vi "process_resistance_arrays.vi"(8 "error in (no error)":errorcluster, 10 "Array":dbl[][](array[numeric]), 11 "TempProbeSet in":refnum<class "TempProbeSet.lvclass">) -> (0 "error out":errorcluster, 3 "TempProbeSet out":refnum<class "TempProbeSet.lvclass">)   [LabVIEW 2010, in "TempProbeSet.lvclass"]
uses:
  TempProbeSet.lvclass
  TempProbe.lvclass
  accessors/read_probes.vi
  accessors/write_probes.vi
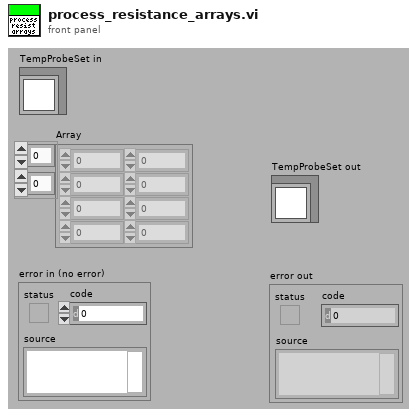
[diagram p1: front panel]
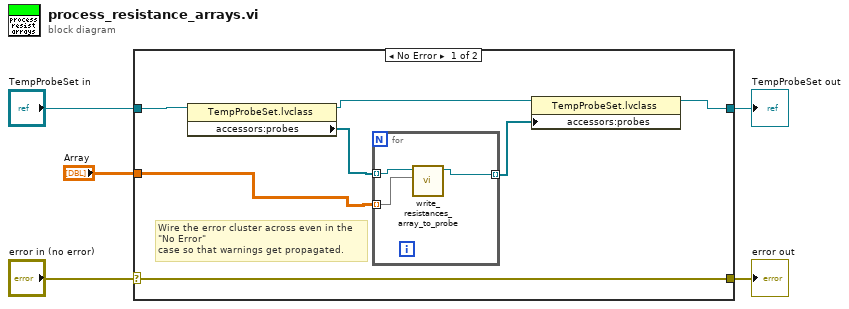
[diagram p0: block diagram]
diagram:
  n1 = case shown="No Error" "error in (no error)" {
    selector: "error in (no error)" -> [w11 w17]
    tunnel: [w11 w17] -> w4
    tunnel: [w7 w16] -> w2
    tunnel: "TempProbeSet in" -> [w12 w16]
    tunnel: "Array" -> [w9 _]
    frame No Error {
      # "Wire the error cluster across even in the \"No Error\"\ncase so that warnings get propagated."
      n2 = property class="TempProbeSet.lvclass"(reference=w12) -> (reference out=w8:refnum<class "TempProbeSet.lvclass">, "accessors:probes"=w10:refnum<class "TempProbe.lvclass">[])  [unwired: 1 in, 1 out]
      n3 = for {
        tunnel: w10 -> [w15] mode=indexing
        tunnel: w9 -> [w14] mode=indexing
        tunnel: [w13] -> w6 mode=indexing
        n4 = call "write_resistances_array_to_probe.vi"("resistances array"=w14, "TempProbe in"=w15) -> ("TempProbe out"=w13:refnum<class "TempProbe.lvclass">)  [unwired: 8 in, 1 out]
      }
      n5 = property class="TempProbeSet.lvclass"(reference=w8, "accessors:probes"=w6) -> (reference out=w7:refnum<class "TempProbeSet.lvclass">)  [unwired: 1 in, 1 out]
    }
    frame Error {
    }
  }
  "error out" <- w4
  "TempProbeSet out" <- w2
